vi "Write Data.vi"(8 "error in (no error)":errorcluster, 10 "Data":T1[](array[typedef]), 11 "bt_Blackboard in":refnum<class "Blackboard.lvclass">) -> (0 "error out":errorcluster, 3 "bt_Blackboard out":refnum<class "Blackboard.lvclass">)   [LabVIEW 2021]
uses:
  Blackboard.lvclass
  Support/Data DVR Type.ctl
  Support/Tags Map Type.ctl
  Support/Status Type.ctl
  Support/Data Type.ctl
  Blackboard.lvclass/Blackboard.ctl
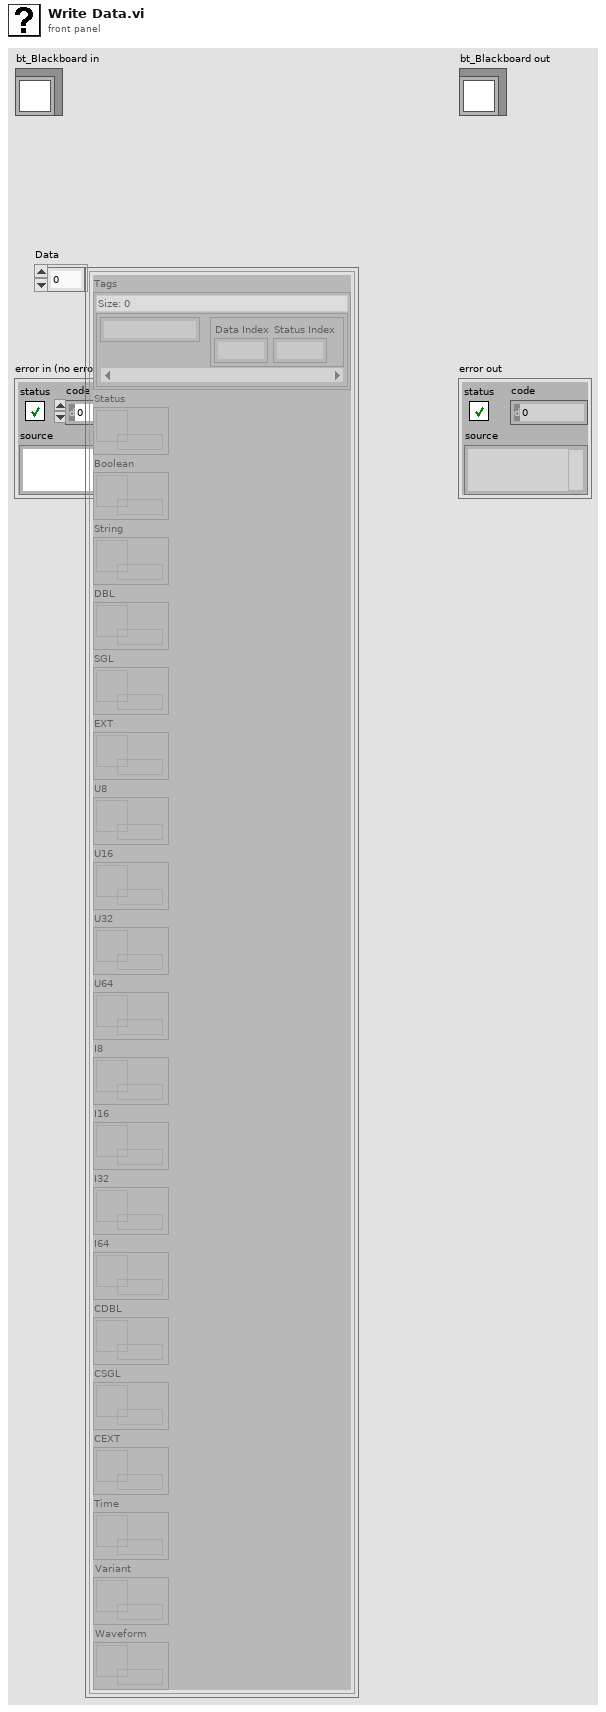
[diagram p1: front panel]
types:
  T1 = typedef "Blackboard.lvclass/Data DVR Type.ctl" = cluster{"Tags":T2, "Status":refnum<data-value>, "Boolean":refnum<data-value>, "String":refnum<data-value>, "DBL":refnum<data-value>, "SGL":refnum<data-value>, "EXT":refnum<data-value>, "U8":refnum<data-value>, "U16":refnum<data-value>, "U32":refnum<data-value>, "U64":refnum<data-value>, "I8":refnum<data-value>, "I16":refnum<data-value>, "I32":refnum<data-value>, "I64":refnum<data-value>, "CDBL":refnum<data-value>, "CSGL":refnum<data-value>, "CEXT":refnum<data-value>, "Time":refnum<data-value>, "Variant":refnum<data-value>, "Waveform":refnum<data-value>}
  T2 = typedef "Blackboard.lvclass/Tags Map Type.ctl" = map{string, cluster{"Data Index":i32, "Status Index":i32}}
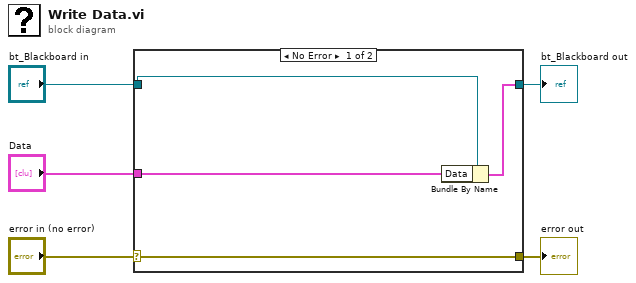
[diagram p0: block diagram]
diagram:
  n1 = case shown="No Error" "error in (no error)" {
    selector: "error in (no error)" -> [w9 w10]
    tunnel: [w9 w10] -> w4
    tunnel: [w7 w11] -> w2
    tunnel: "bt_Blackboard in" -> [w8 w11]
    tunnel: "Data" -> [w6 _]
    frame No Error {
      n2 = Bundle By Name(cluster=w8, "Data"=w6) -> (w7:cluster{})
    }
    frame Error {
    }
  }
  "error out" <- w4
  "bt_Blackboard out" <- w2
